vi "Create RT queues.vi"() -> (3 "Queues":T1)   [LabVIEW 2018]
doc: "Create the Queues required for the Compressor Rig RT application:\n\nMessage queue (string + variant)\nAnalogue data (double array)\nTorque data (double array)\n\nAfter initialisation an 'init' message is written to the RT Message queue"
uses:
  Type Defs/Queues cluster.ctl
  ICL-LabVIEW_General/Message Scheduler/message scheduler.lvclass
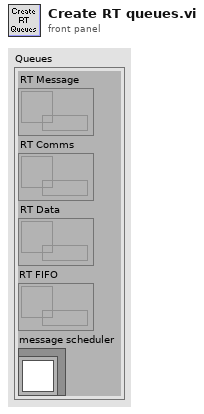
[diagram p1: front panel]
types:
  T1 = typedef "Queues cluster.ctl" = cluster{"RT Message":refnum<queue>, "RT Comms":refnum<queue>, "RT Data":refnum<queue>, "RT FIFO":refnum<queue>, "message scheduler":refnum<class "message scheduler.lvclass">}
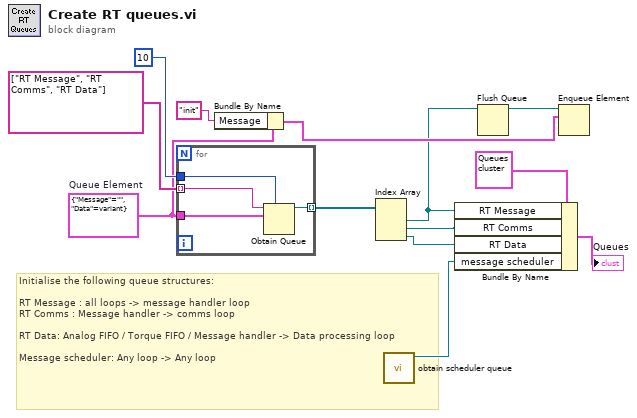
[diagram p0: block diagram]
diagram:
  w7 = cluster{"Message":string, "Data":variant} {"Message"="", "Data"=variant}  # Queue Element
  # "Initialise the following queue structures:\n\nRT Message : all loops -> message handler loop\nRT Comms : Message handler -> comms loop\n\nRT Data: Analog FIFO / Torque FIFO / Message handler -> Data processing loop\n\nMessage scheduler: Any loop -> Any loop"
  n1 = for {
    tunnel: string[] ["RT Message", "RT Comms", "RT Data"] ("name (unnamed)") -> [w17] mode=indexing
    tunnel: 10 ("max queue size (-1, unlimited)") -> [w16]
    tunnel: [w15] -> w9 mode=indexing
    tunnel: w7 -> [w14]
    n2 = Obtain Queue(max queue size (-1, unlimited)=w16, name (unnamed)=w17, element data type=w14) -> (queue out=w15:refnum<queue>)  [unwired: 2 in, 2 out]
  }
  n3 = Bundle By Name(cluster=w7, "Message"="init") -> (w10:cluster{"Message":string, "Data":variant})
  n4 = Index Array(array=w9) -> (element #1=w4:refnum<queue>, element #2=w3:refnum<queue>, element #3=w1:refnum<queue>)  [unwired: 3 in]
  n5 = call "obtain scheduler queue.vi"() -> ("message scheduler out"=w2:refnum<class "message scheduler.lvclass">)  [unwired: 10 in, 1 out]
  n6 = Bundle By Name(cluster=T1 {"RT Message"=refnum, "RT Comms"=refnum, "RT Data"=refnum, "RT FIFO"=refnum, "message scheduler"=refnum} ("RT Queues"), "RT Message"=w4, "RT Comms"=w3, "RT Data"=w1, "message scheduler"=w2) -> (→"Queues":T1)
  n7 = Flush Queue(queue=w4) -> (queue out=w8:refnum<queue>)  [unwired: 1 in, 2 out]
  n8 = Enqueue Element(queue=w8, element=w10) -> ()  [unwired: 2 in, 3 out]
